vi "Humidity Server.vi"   [LabVIEW 2012]
uses:
  <vilib>/DAQmx/read.llb/DAQmx Read (Analog 2D DBL NChan NSamp).vi
  <vilib>/DAQmx/write.llb/DAQmx Write (Digital 1D Bool NChan 1Samp 1Line).vi
  <vilib>/DAQmx/write.llb/DAQmx Write (Analog 1D DBL NChan 1Samp).vi
  Reusable/Serial IO/Serial IO.lvclass
  <vilib>/DAQmx/write.llb/DAQmx Write (Analog DBL 1Chan 1Samp).vi
  <vilib>/Analysis/NI_AALBase.lvlib
  <vilib>/Analysis/baseanly.llb/Mean (DBL).vi
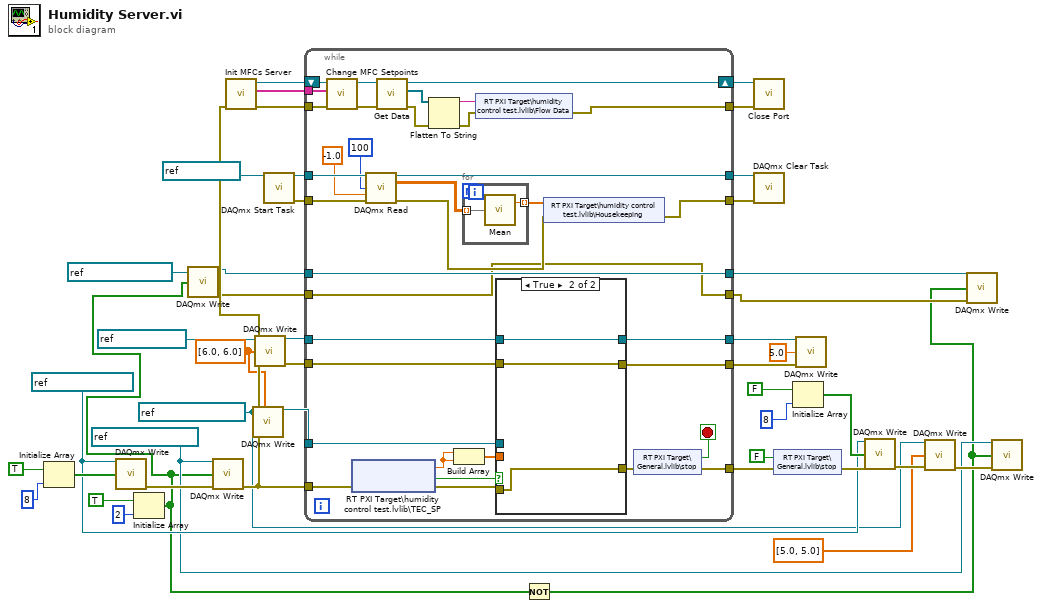
[diagram p0: block diagram]
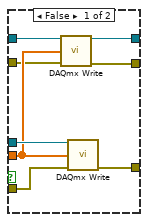
[diagram p2: hidden frame]
diagram:
  w1 = dbl[] [6.0, 6.0] ("data")
  w22 = refnum<k21> "PS Switch Out" ("task/channels in")
  w18 = refnum<k21> "CRD Hum T En" ("task/channels in")
  w3 = refnum<k21> "CRD Hum T SP" ("task/channels in")
  n1 = Initialize Array(TRUE, 8 ("dimension size")) -> (w43:bool[])
  n2 = call-poly <vilib>:"DAQmx Write.vi"("task/channels in"=w22, "data"=w43) -> ("error out"=w39:errorcluster)  [unwired: 11 in, 2 out]
  n3 = Initialize Array(TRUE, 2 ("dimension size")) -> (w8:bool[])
  n4 = call-poly <vilib>:"DAQmx Write.vi"("task/channels in"=refnum<k21> "PAS Hum T En", "data"=w8) -> ("task out"=w12:refnum<k21>, "error out"=w10:errorcluster)  [unwired: 11 in, 1 out]
  n5 = call-poly <vilib>:"DAQmx Write.vi"("task/channels in"=w18, "data"=w8, "error in"=w39) -> ("error out"=w17:errorcluster)  [unwired: 10 in, 2 out]
  n6 = call "Init MFCs Server.vi"("error in"=w17) -> ("error out"=w29:errorcluster, "Address Out"=w30:string[], "Serial IO out"=w31:refnum<class "Serial IO.lvclass">)  [unwired: 8 in]
  n7 = call-poly <vilib>:"DAQmx Write.vi"("task/channels in"=w3, "data"=w1) -> ("task out"=w2:refnum<k21>)  [unwired: 11 in, 2 out]
  n8 = call-poly <vilib>:"DAQmx Write.vi"("task/channels in"=refnum<k21> "PAS TEC SP", "data"=w1) -> ("task out"=w5:refnum<k21>, "error out"=w4:errorcluster)  [unwired: 11 in, 1 out]
  n9 = call <vilib>:"DAQmx Start Task.vi"("task/channels in"=refnum<k21> "CRD LFIO") -> ("task out"=w35:refnum<k21>, "error out"=w34:errorcluster)  [unwired: 13 in]
  n10 = while {
    tunnel: w35 -> [w78]
    tunnel: [w75] -> w33
    tunnel: w2 -> [w70]
    tunnel: w17 -> [w53]
    tunnel: [w68] -> w37
    tunnel: [w67] -> w32
    tunnel: w34 -> [w66]
    tunnel: w30 -> [w63]
    tunnel: w29 -> [w62]
    shift-right: [w59] -> w28
    shift-left: w31 -> [w64]
    tunnel: [w54] -> w27
    tunnel: w5 -> [w51]
    tunnel: [w49] -> w16
    tunnel: [w48] -> w15
    tunnel: [w47] -> w11
    tunnel: w12 -> [w47]
    tunnel: [w46] -> w9
    tunnel: w10 -> [w46]
    tunnel: w4 -> [w45]
    stop <- w79 stop-if-true
    n11 = call "Change MFC Setpoints.vi"("error in"=w62, "Address Out"=w63, "Serial IO in"=w64) -> ("error out"=w60:errorcluster, "Serial IO Out"=w61:refnum<class "Serial IO.lvclass">)  [unwired: 7 in]
    n12 = shared-variable "RT PXI Target\\humidity control test.lvlib\\TEC_SP"(error in=w53) -> (w50:dbl, error out=w52:errorcluster, w71:bool)  [unwired: 1 in]
    n13 = call-poly <vilib>:"DAQmx Read.vi"("task/channels in"=w78, "number of samples per channel"=100, "timeout"=-1.0, "error in"=w66) -> ("task out"=w75:refnum<k21>, "data"=w74:dbl[][], "error out"=w72:errorcluster)  [unwired: 9 in]
    n14 = call-dynamic "Get Data.vi"("error in (no error)"=w60, "Serial IO in"=w61) -> ("error out"=w57:errorcluster, "DataArray"=w58:refnum<class "Data.lvclass">[], "Serial IO out"=w59:refnum<class "Serial IO.lvclass">)  [unwired: 7 in]
    n15 = Flatten To String(anything=w58, error in (no error)=w57) -> (data string=w56:string, error out=w55:errorcluster)  [unwired: 2 in, 1 out]
    n16 = Build Array(w50, w50) -> (w69:dbl[])
    n17 = for {
      tunnel: w74 -> [w92] mode=indexing
      tunnel: [w91] -> w73 mode=indexing
      n18 = call-poly <vilib>:"Mean.vi"("X"=w92) -> ("mean"=w91:dbl)  [unwired: 1 out]
    }
    n19 = shared-variable "RT PXI Target\\humidity control test.lvlib\\Flow Data"(w56, error in=w55) -> (error out=w54:errorcluster)
    n20 = case shown="True" w71 {
      tunnel: w69 -> [w81 _]
      tunnel: w70 -> [w87 _]
      tunnel: w52 -> [w86 w90]
      tunnel: [w85 w90] -> w65
      tunnel: w51 -> [w84 w89]
      tunnel: [w83 w89] -> w49
      tunnel: [w82 w88] -> w48
      tunnel: w45 -> [w80 w88]
      frame False {
        n21 = call-poly <vilib>:"DAQmx Write.vi"("task/channels in"=w84, "data"=w81, "error in"=w80) -> ("task out"=w83:refnum<k21>, "error out"=w82:errorcluster)  [unwired: 10 in, 1 out]
        n22 = call-poly <vilib>:"DAQmx Write.vi"("task/channels in"=w87, "data"=w81, "error in"=w86) -> ("error out"=w85:errorcluster)  [unwired: 10 in, 2 out]
      }
      frame True {
      }
    }
    n23 = shared-variable "RT PXI Target\\humidity control test.lvlib\\Housekeeping"(w73, error in=w72) -> (error out=w67:errorcluster)
    n24 = shared-variable "RT PXI Target\\General.lvlib\\stop"(error in=w65) -> (w79:bool, error out=w68:errorcluster)
  }
  n25 = Not(x=w8) -> (.not. x?=w7:bool[])
  n26 = call-dynamic "Close Port.vi"("error in (no error)"=w27, "Serial IO in"=w28) -> ()  [unwired: 8 in, 2 out]
  n27 = call <vilib>:"DAQmx Clear Task.vi"("task in"=w33, "error in"=w32) -> ()  [unwired: 13 in, 1 out]
  n28 = shared-variable "RT PXI Target\\General.lvlib\\stop"(FALSE ("stop"), error in=w37) -> (error out=w24:errorcluster)
  n29 = Initialize Array(FALSE, 8 ("dimension size")) -> (w26:bool[])
  n30 = call-poly <vilib>:"DAQmx Write.vi"("task/channels in"=w16, "data"=5.0, "error in"=w15) -> ()  [unwired: 10 in, 3 out]
  n31 = call-poly <vilib>:"DAQmx Write.vi"("task/channels in"=w22, "data"=w26, "error in"=w24) -> ("error out"=w21:errorcluster)  [unwired: 10 in, 2 out]
  n32 = call-poly <vilib>:"DAQmx Write.vi"("task/channels in"=w3, "data"=dbl[] [5.0, 5.0], "error in"=w21) -> ("error out"=w19:errorcluster)  [unwired: 10 in, 2 out]
  n33 = call-poly <vilib>:"DAQmx Write.vi"("task/channels in"=w11, "data"=w7, "error in"=w9) -> ()  [unwired: 10 in, 3 out]
  n34 = call-poly <vilib>:"DAQmx Write.vi"("task/channels in"=w18, "data"=w7, "error in"=w19) -> ()  [unwired: 10 in, 3 out]
